vi "Auto settings.vi"(8 "error in (no error)":errorcluster, 10 "Array":dbl[](array[numeric]), 11 "Syringe Space in":refnum<class "Syringe Space.lvclass">) -> (0 "error out":errorcluster, 3 "Syringe Space out":refnum<class "Syringe Space.lvclass">)   [LabVIEW 2021, in "Syringe Space.lvclass"]
uses:
  Syringe Space.lvclass
  C:/Users/HEP/Documents/GitHub/UCSB-Gantry-HEP/Classes/Workspace/Fixture.lvclass
  C:/Users/HEP/Documents/GitHub/UCSB-Gantry-HEP/Classes/Workspace/Carrier Tray/Assembly Tray.lvclass
  Fixture.lvclass/Fixture.ctl
  Assembly Tray.lvclass/Assembly Tray.ctl
  Write Fixture ID.vi
  Write Syringe.vi
  Write Gantry Region.vi
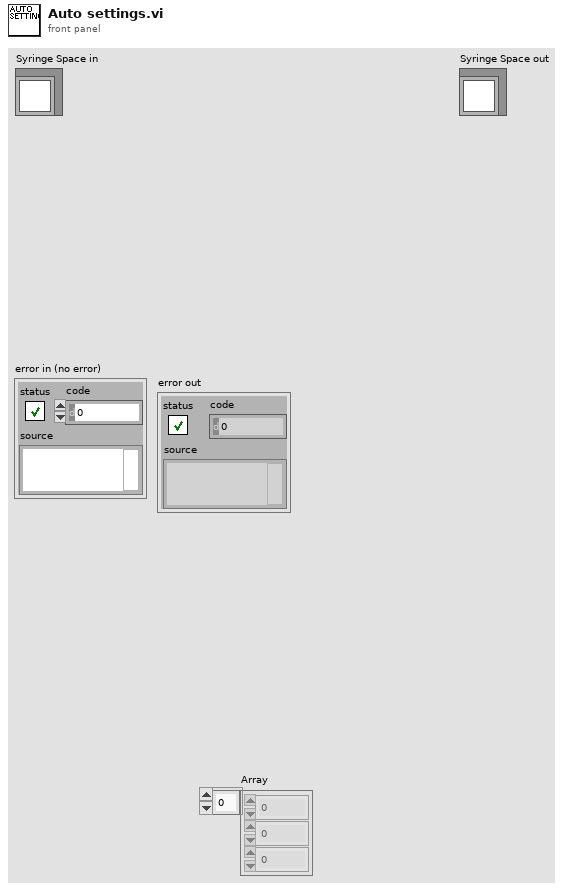
[diagram p1: front panel]
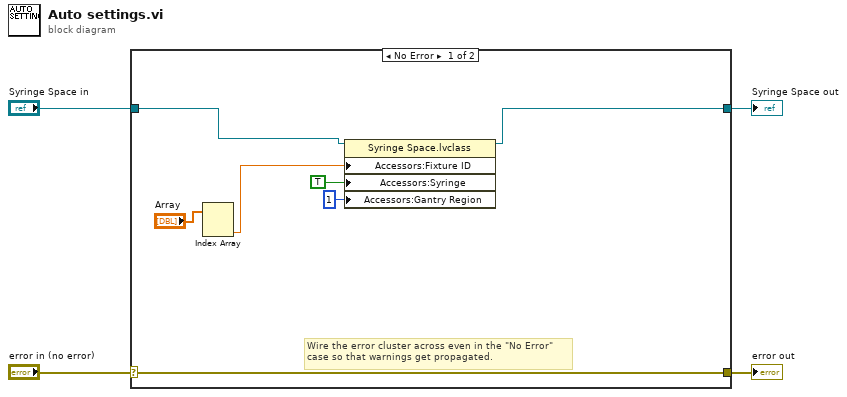
[diagram p0: block diagram]
diagram:
  n1 = case shown="No Error" "error in (no error)" {
    selector: "error in (no error)" -> [w11 w13]
    tunnel: [w11 w13] -> w3
    tunnel: [w8 w12] -> w1
    tunnel: "Syringe Space in" -> [w9 w12]
    frame No Error {
      # "Wire the error cluster across even in the \"No Error\"\ncase so that warnings get propagated."
      n2 = Index Array(array="Array") -> (element #2=w6:dbl)  [unwired: 2 in, 1 out]
      n3 = property class="Syringe Space.lvclass"(reference=w9, "Accessors:Fixture ID"=w6, "Accessors:Syringe"=TRUE ("Syringe"), "Accessors:Gantry Region"=1 ("Gantry Region")) -> (reference out=w8:refnum<class "Syringe Space.lvclass">)  [unwired: 1 in, 1 out]
    }
    frame Error {
    }
  }
  "error out" <- w3
  "Syringe Space out" <- w1
